vi "Lookup Fault Code.vi"(8 "error in (no error)":errorcluster, 11 "FaultCode":i32) -> (0 "error out":errorcluster, 1 "Fault":bool, 2 "Description":string, 3 "Fault Bits":bool[](array[boolean]))   [LabVIEW 2021]
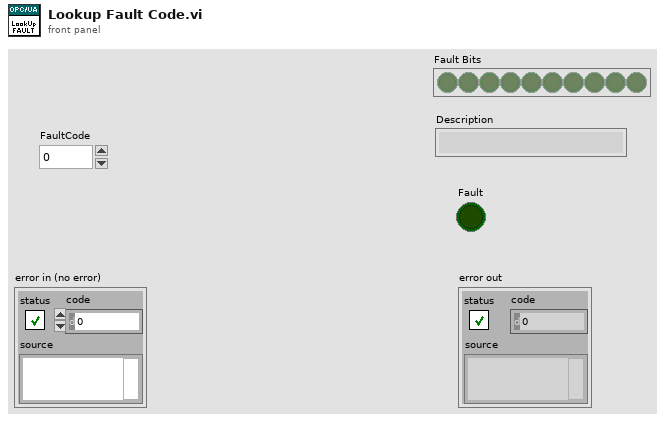
[diagram p1: front panel]
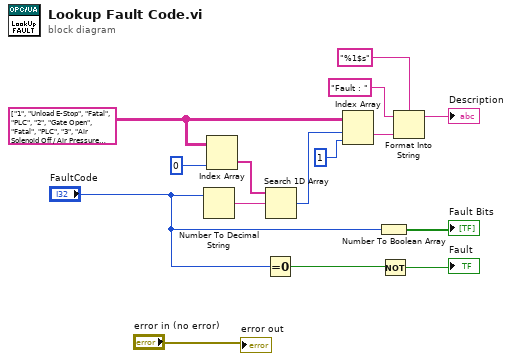
[diagram p0: block diagram]
diagram:
  w10 = string[][] [["1", "Unload E-Stop", "Fatal", "PLC"], ["2", "Gate Open", "Fatal", "PLC"], ["3", "Air Solenoid Off / Air Pressure Low", "Fatal", "PLC"], ["8", "Clamp Fault", "Error", "PLC"], ["9", "Left Terminal Cylinder Fault", "Error", "PLC"], ["10", "Hioki Cylinder Fault", "Error", "PLC"], ["11", "Center Terminal Cylinder Fault", "Error", "PLC"], ["12", "Right Terminal Cylinder Fault", "Error", "PLC"], ["16", "Timeout Fault", "Warning", "PLC"]]
  n1 = Number To Decimal String(number="FaultCode") -> (decimal integer string=w6:string)  [unwired: 1 in]
  n2 = Index Array(array=w10, index (col)=0 ("disabled index (col)")) -> (element=w7:string[])  [unwired: 1 in]
  n3 = Equal To 0?(x="FaultCode") -> (x = 0?=w9:bool)
  n4 = Search 1D Array(1D array=w7, element=w6) -> (index of element=w8:i32)  [unwired: 1 in]
  n5 = Index Array(array=w10, index (row)=w8, index (col)=1 ("disabled index (col)")) -> (element=w5:string)
  n6 = Number To Boolean Array(number="FaultCode") -> (Boolean array=→"Fault Bits":bool[])
  n7 = Not(x=w9) -> (.not. x?=→"Fault":bool)
  n8 = Format Into String(format string="%1$s", initial string="Fault : ", w5) -> (resulting string=→"Description":string)  [unwired: 1 in, 1 out]
  "error out" <- "error in (no error)"
